vi "Decode Internal Text.vi"(8 "error in (no error)":errorcluster, 11 "data":u8[](array[numeric])) -> (0 "error out":errorcluster, 3 "string":string)   [LabVIEW 2020, in "NI_SFTP.lvlib"]
uses:
  <vilib>/net/SFTP/NI_SFTP.lvlib
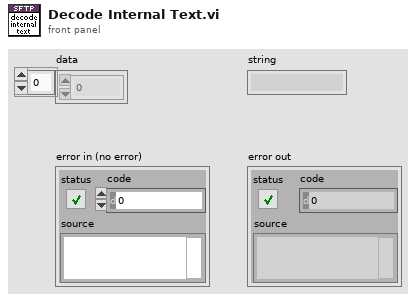
[diagram p1: front panel]
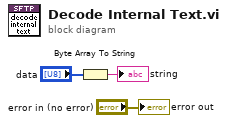
[diagram p0: block diagram]
diagram:
  n1 = Byte Array To String(unsigned byte array="data") -> (string=→"string":string)
  "error out" <- "error in (no error)"
